vi "find avg of n size array.vi"() -> ()   [LabVIEW 2012]
panel:
  out "sum":dbl
  out "x/y":dbl
  out "product":i32
  out "size(s)":i32[](array[numeric])
  out "Array":dbl[][](array[numeric])
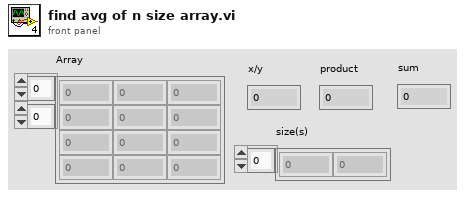
[diagram p1: front panel]
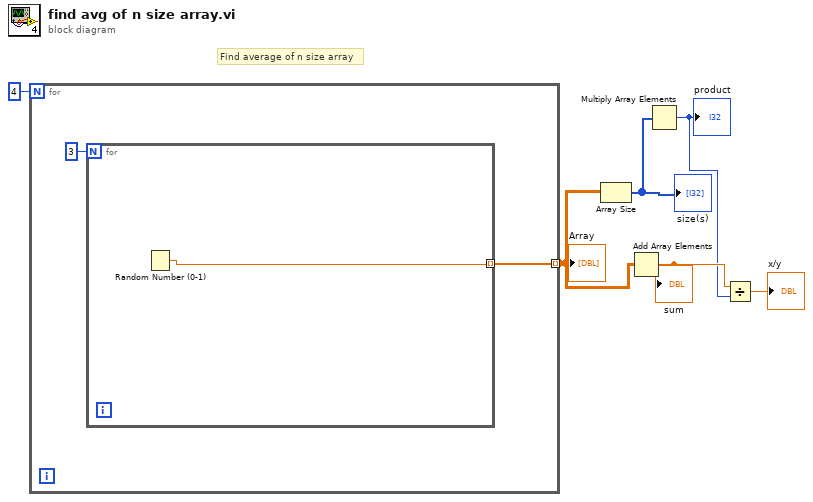
[diagram p0: block diagram]
diagram:
  # "Find average of n size array"
  n1 = for {
    N: 4 -> [_]
    tunnel: [w7] -> w5 mode=indexing
    n2 = for {
      N: 3 -> [_]
      tunnel: [w9] -> w7 mode=indexing
      n3 = Random Number (0-1)() -> (number: 0 to 1=w9:dbl)
    }
  }
  "Array" <- w5
  n4 = Array Size(array=w5) -> (size(s)=w4:i32[])
  "size(s)" <- w4
  n5 = Add Array Elements(numeric array=w5) -> (sum=w3:dbl)
  "sum" <- w3
  n6 = Multiply Array Elements(1:w4) -> (0:w2:i32)
  "product" <- w2
  n7 = Divide(x=w3, y=w2) -> (x/y=→"x/y":dbl)
